vi "Outputs SW Set.vi"(7 "CMD Data":T5 {"Auto Angle" scale format="%.3f"; "Direction"."Rotate(Yaw) CCW 1 CW -1" scale=1.0..-1.0; "Direction"."Traverse"."Angle" scale format="%.3f"; "Direction"."Traverse"."Velocity" scale=-1.0..1.0 scale format="%.1f"}, 8 "Auto Rotate PID":T2 {"Max I Accu"."Low" format="%#.8f"; "Max I Accu"."High" format="%#.8f"; "Gains"."F" format="%#.8f"; "Gains"."D" format="%#.8f"; "Gains"."I" format="%#.8f"; "Gains"."P" format="%#.8f"; "Error Allowed"."Low" format="%#.8f"; "Error Allowed"."High" format="%#.8f"; "I Zone"."Low" format="%#.8f"; "I Zone"."High" format="%#.8f"; "Peak Out 0-1"."Low" format="%#.8f"; "Peak Out 0-1"."High" format="%#.8f"}, 10 "Compass Heading":T10 scale format="%.3f", 11 "System Output Data":T1) -> (3 "System Output Data Out":T1, 5 "CMD Data Out":T5 {"Auto Angle" scale format="%.3f"; "Direction"."Rotate(Yaw) CCW 1 CW -1" scale=1.0..-1.0; "Direction"."Traverse"."Angle" scale format="%.3f"; "Direction"."Traverse"."Velocity" scale=-1.0..1.0 scale format="%.1f"})   [LabVIEW 2023, in "SwerveDrive_ACT_ts.lvlib"]
uses:
  SwerveDrive_ACT_ts.lvlib
  182fe2e2-5080-48b1-a7d8-08075c65323e.vi
  Shared Code/TypeDefs/Dial_Compase heading unit circle CCW positive.ctl
  Shared Code/TypeDefs/Level_Velocity plus-minus 1.ctl
  Shared Code/TypeDefs/Cluster_Module Velocity-Direction-Rotations.ctl
  Shared Code/TypeDefs/Cluster_CMD_Direction Data.ctl
  Shared Code/TypeDefs/Cluster_X-Y.ctl
  Shared Code/TypeDefs/ENUM_CMD_Mode Select.ctl
  Cluster_CMD_ACT_Data.ctl
  Shared Code/TypeDefs/Cluster_High-Low.ctl
  Shared Code/TypeDefs/Cluster_PID Gains.ctl
  Shared Code/TypeDefs/Cluster_SW PID Config.ctl
  Cluster_System Output Data.ctl
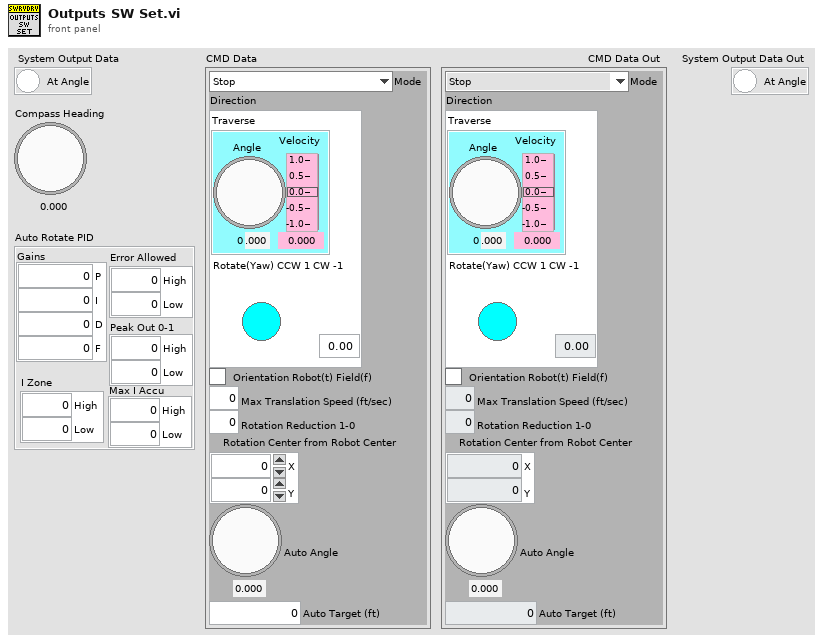
[diagram p1: front panel]
types:
  T1 = typedef "SwerveDrive_ACT_ts.lvlib/Cluster_System Output Data.ctl" = cluster{"At Angle":bool}
  T2 = typedef "Cluster_SW PID Config.ctl" = cluster{"Gains":T3, "Error Allowed":T4, "I Zone":T4, "Peak Out 0-1":T4, "Max I Accu":T4}
  T3 = typedef "Cluster_PID Gains.ctl" = cluster{"P":dbl, "I":dbl, "D":dbl, "F":dbl}
  T4 = typedef "Cluster_High-Low.ctl" = cluster{"High":dbl, "Low":dbl}
  T5 = typedef "SwerveDrive_ACT_ts.lvlib/Cluster_CMD_ACT_Data.ctl" = cluster{"Mode":T6, "Direction":T7, "Orientation Robot(t) Field(f)":bool, "Max Translation Speed (ft/sec)":dbl, "Rotation Reduction 1-0":dbl, "Rotation Center from Robot Center":T11, "Auto Angle":T10, "Auto Target (ft)":dbl}
  T6 = typedef "ENUM_CMD_Mode Select.ctl" = enum16{"Stop", "Translate Cmd Rotate Cmd", "Translate Cmd Rotate Auto"}
  T7 = typedef "Cluster_CMD_Direction Data.ctl" = cluster{"Traverse":T8, "Rotate(Yaw) CCW 1 CW -1":dbl}
  T8 = typedef "Cluster_Module Velocity-Direction-Rotations.ctl" = cluster{"Velocity":T9, "Angle":T10, "Rotations Count":dbl}
  T9 = typedef "Level_Velocity plus-minus 1.ctl" = dbl
  T10 = typedef "Dial_Compase heading unit circle CCW positive.ctl" = dbl
  T11 = typedef "Cluster_X-Y.ctl" = cluster{"X":dbl, "Y":dbl}
  T12 = typedef "NUM_Rotate Input.ctl" = dbl
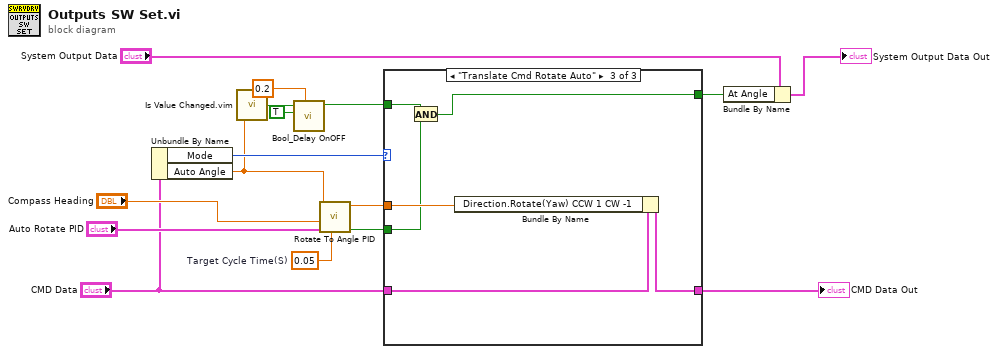
[diagram p0: block diagram]
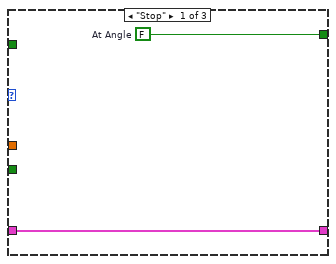
[diagram p2: hidden frame]
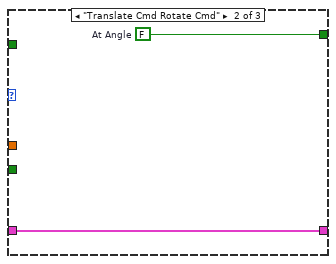
[diagram p3: hidden frame]
diagram:
  w14 = 0.05  # Target Cycle Time(S)
  n1 = Unbundle By Name("CMD Data") -> ("Mode"=w11:T6, "Auto Angle"=w2:T10)
  n2 = call "Is Value Changed.vim"("value"=w2) -> ("changed or first call?"=w5:bool)
  n3 = call "Bool_Delay OnOFF.vi"("Delay Time(S)"=0.2, "Delay On(t) Off(f)"=TRUE, "Input"=w5) -> ("Output"=w1:bool)  [unwired: 7 in, 1 out]
  n4 = call "Rotate To Angle PID.vi"("Target Cycle Time(S)"=w14, "PID Config"="Auto Rotate PID", "Current Yaw"="Compass Heading", "Target Yaw"=w2) -> ("At Angle Out"=w6:bool, "Direction.Rotate(Yaw) CCW 1 CW -1 Out"=w7:T12)  [unwired: 5 in, 1 out]
  n5 = case shown="\"Translate Cmd Rotate Auto\"" w11 {
    tunnel: "CMD Data" -> [w17 w19 w26]
    tunnel: [w17 w19 w25] -> w12
    tunnel: [w18 w20 w22] -> w9
    tunnel: w7 -> [_ _ w24]
    tunnel: w6 -> [_ _ w21]
    tunnel: w1 -> [_ _ w23]
    frame "Stop" {
      w18 = FALSE  # At Angle
    }
    frame "Translate Cmd Rotate Cmd" {
      w20 = FALSE  # At Angle
    }
    frame "Translate Cmd Rotate Auto" {
      n6 = And(x=w23, y=w21) -> (x .and. y?=w22:bool)
      n7 = Bundle By Name(cluster=w26, "Direction.Rotate(Yaw) CCW 1 CW -1"=w24) -> (w25:T5)
    }
  }
  "CMD Data Out" <- w12
  n8 = Bundle By Name(cluster="System Output Data", "At Angle"=w9) -> (→"System Output Data Out":T1)
